vi "ma_Tone estimation subroutine G(f) (FFT input).vi"(4 "N (window length)":i32=512, 5 "window":u16(ring) items=["Rectangle"=0, "Hanning"=1, "Hamming"=2, "Blackman-Harris"=3, "Exact Blackman"=4, "Blackman"=5, "Flat Top"=6, "4 Term B-Harris "=7, "7 Term B-Harris"=8, "Low Sidelobe"=9, "Blackman Nuttall"=11, "Triangle"=30, "Bartlett-Hanning"=31, "Bohman"=32, "Parzen"=33, "Welch"=34, "Kaiser"=60, "Dolph-Chebyshev"=61, "Gaussian"=62], 6 "frequency":dbl format="%.5e", 7 "three fingers":T1={"f0"=0.0, "df"=1.0, "spectrum"=[]} {"spectrum" format="%.2f"; "df" format="%.2f"; "f0" format="%.2f"}) -> (1 "phase [degree]":dbl format="%.2f", 2 "Amplitude":dbl format="%.2f", 3 "G(f)":dbl format="%.2e")   [LabVIEW 2020, in "NI_MAPro.lvlib"]
doc: "This is the actual function involved in the Newton-Raphson's root finding loop.\nG(f) is the function to be evaluated. for each iteration, amplitude and phase are also computed."
uses:
  NI_MAPro.lvlib
  ma_sml_Spectrum Cluster (complex).ctl
  NI_AALBase.lvlib
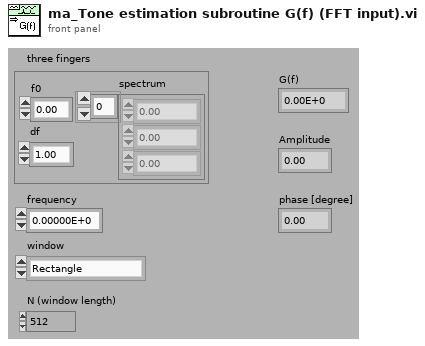
[diagram p1: front panel]
types:
  T1 = typedef "NI_MAPro.lvlib/ma_sml_Spectrum Cluster (complex).ctl" = cluster{"f0":dbl, "df":dbl, "spectrum":cdb[]}
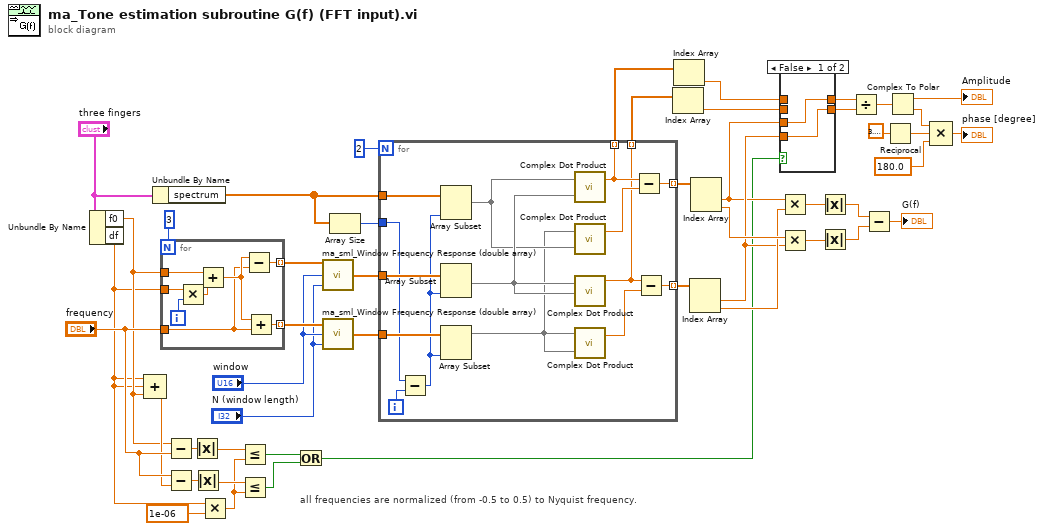
[diagram p0: block diagram]
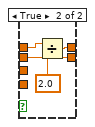
[diagram p2: hidden frame]
diagram:
  # "all frequencies are normalized (from -0.5 to 0.5) to Nyquist frequency."
  n1 = Unbundle By Name("three fingers") -> ("f0"=w4:dbl, "df"=w3:dbl)
  n2 = Compound Arithmetic op=ADD(w3, w3, w4) -> (w23:dbl)
  n3 = Unbundle By Name("three fingers") -> ("spectrum"=w5:cdb[])
  n4 = for {
    N: 3 -> [_]
    tunnel: w4 -> [w56]
    tunnel: w3 -> [w53]
    tunnel: "frequency" -> [w51]
    tunnel: [w50] -> w39 mode=indexing
    tunnel: [w49] -> w38 mode=indexing
    i -> [w54]
    n5 = Multiply(x=w53, y=w54) -> (x*y=w55:dbl)
    n6 = Add(x=w56, y=w55) -> (x+y=w52:dbl)
    n7 = Subtract(x=w52, y=w51) -> (x-y=w50:dbl)
    n8 = Add(x=w52, y=w51) -> (x+y=w49:dbl)
  }
  n9 = Subtract(x=w4, y="frequency") -> (x-y=w22:dbl)
  n10 = Subtract(x="frequency", y=w23) -> (x-y=w21:dbl)
  n11 = Absolute Value(x=w22) -> (abs(x)=w20:dbl)
  n12 = Absolute Value(x=w21) -> (abs(x)=w19:dbl)
  n13 = Multiply(x=w3, y=1e-06) -> (x*y=w1:dbl)
  n14 = Less Or Equal?(x=w20, y=w1) -> (x <= y?=w18:bool)
  n15 = Less Or Equal?(x=w19, y=w1) -> (x <= y?=w8:bool)
  n16 = Or(x=w18, y=w8) -> (x .or. y?=w7:bool)
  n17 = call "ma_sml_Window Frequency Response (double array).vi"("N (window length)"="N (window length)", "window"="window", "f(normalized)"=w39) -> ("H(f)"=w35:cdb[])
  n18 = call "ma_sml_Window Frequency Response (double array).vi"("N (window length)"="N (window length)", "window"="window", "f(normalized)"=w38) -> ("H(f)"=w36:cdb[])
  n19 = Array Size(array=w5) -> (size(s)=w29:i32)
  n20 = for {
    N: 2 -> [_]
    tunnel: w5 -> [w71]
    tunnel: w36 -> [w69]
    tunnel: w35 -> [w70]
    tunnel: [w66] -> w33 mode=indexing
    tunnel: [w63] -> w32 mode=indexing
    tunnel: w29 -> [w64]
    tunnel: [w62] -> w13 mode=indexing
    tunnel: [w61] -> w12 mode=indexing
    i -> [w60]
    n21 = Subtract(x=w64, y=w60) -> (x-y=w65:i32)
    n22 = Array Subset(array=w71, length=w65) -> (w58:cdb[])  [unwired: 1 in]
    n23 = Array Subset(array=w70, length=w65) -> (w59:cdb[])  [unwired: 1 in]
    n24 = Array Subset(array=w69, length=w65) -> (w57:cdb[])  [unwired: 1 in]
    n25 = call "Complex Dot Product.vi"("Y Vector"=w59, "X Vector"=w58) -> ("X * Y"=w62:cdb)  [unwired: 1 out]
    n26 = call "Complex Dot Product.vi"("Y Vector"=w58, "X Vector"=w57) -> ("X * Y"=w68:cdb)  [unwired: 1 out]
    n27 = call "Complex Dot Product.vi"("Y Vector"=w59, "X Vector"=w59) -> ("X * Y"=w61:cdb)  [unwired: 1 out]
    n28 = call "Complex Dot Product.vi"("Y Vector"=w57, "X Vector"=w57) -> ("X * Y"=w67:cdb)  [unwired: 1 out]
    n29 = Subtract(x=w62, y=w68) -> (x-y=w66:cdb)
    n30 = Subtract(x=w61, y=w67) -> (x-y=w63:cdb)
  }
  n31 = Index Array(array=w12) -> (element=w11:cdb)  [unwired: 1 in]
  n32 = Index Array(array=w13) -> (element=w10:cdb)  [unwired: 1 in]
  n33 = Index Array(array=w32) -> (element #1=w17:cdb, element #2=w26:cdb)  [unwired: 2 in]
  n34 = Index Array(array=w33) -> (element #1=w15:cdb, element #2=w27:cdb)  [unwired: 2 in]
  n35 = case shown="False" w7 {
    tunnel: w17 -> [w73 _]
    tunnel: [w73 w76] -> w16
    tunnel: w15 -> [w72 _]
    tunnel: [w72 w75] -> w14
    tunnel: w10 -> [_ w77]
    tunnel: w11 -> [_ w76]
    frame False {
    }
    frame True {
      n36 = Divide(x=w77, y=2.0) -> (x/y=w75:cdb)
    }
  }
  n37 = Multiply(x=w15, y=w26) -> (x*y=w31:cdb)
  n38 = Multiply(x=w27, y=w17) -> (x*y=w30:cdb)
  n39 = Absolute Value(x=w31) -> (abs(x)=w47:dbl)
  n40 = Absolute Value(x=w30) -> (abs(x)=w46:dbl)
  n41 = Divide(x=w14, y=w16) -> (x/y=w25:cdb)
  n42 = Subtract(x=w47, y=w46) -> (x-y=→"G(f)":dbl)
  n43 = Reciprocal(x=3.141592653589793) -> (1/x=w43:dbl)
  n44 = Complex To Polar(r * e^(i*theta)=w25) -> (r=→"Amplitude":dbl, theta=w45:dbl)
  n45 = Compound Arithmetic op=MULTIPLY(w45, w43, 180.0 ("Input")) -> (→"phase [degree]":dbl)
